vi "RSNRPZ Initialize Z5.vi"(8 "error in (no error)":errorcluster, 9 "Reset Device (T: Reset Device)":bool=TRUE, 10 "ID Query (T: Do Query)":bool=TRUE, 11 "Port (A)":i32(ring) items=["A", "B", "C", "D"]) -> (0 "error out":errorcluster, 2 "Function return value":i32, 3 "Instrument Handle":u32)   [LabVIEW 2010]
doc: "This VI performs the following initialization actions and assigned specified sesnor to channel 1:\n\n- Opens a session to the specified device using the interface and address specified in the Resource Name control.\n\n- Performs an identification query on the sensor.\n\n- Resets the instrument to a known state.\n\n- Sends initialization commands to the sensor\n\n- Returns an Instrument Handle which is used to differentiate between different sessions of this instrument driver."
uses:
  rsnrpz_32.dll
panel:
  # "Warning: The driver requires NRP Toolkit installed on your computer"
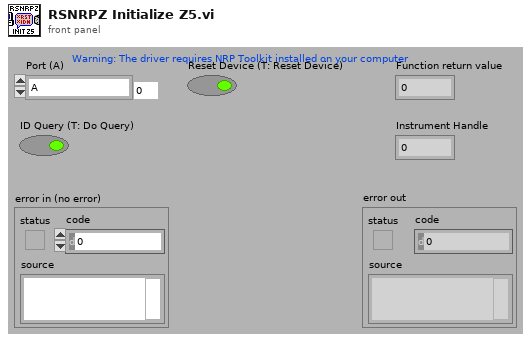
[diagram p1: front panel]
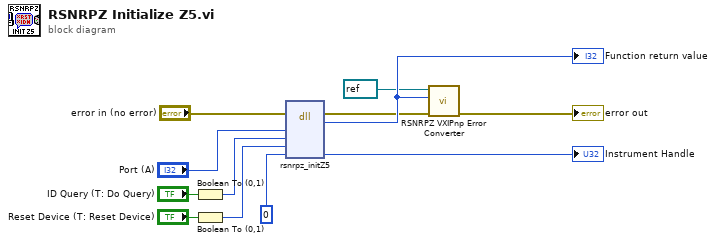
[diagram p0: block diagram]
diagram:
  n1 = Boolean To (0,1)(Boolean="ID Query (T: Do Query)") -> (0, 1=w8:i16)
  n2 = Boolean To (0,1)(Boolean="Reset Device (T: Reset Device)") -> (0, 1=w9:i16)
  n3 = dll-call lib="rsnrpz_32.dll" fn="rsnrpz_initZ5"(error in="error in (no error)", "Port"="Port (A)", "ID Query"=w8, "Reset Device"=w9, "Instrument Handle"=u32 0) -> (error out=w3:errorcluster, "return type"=w5:i32, "Instrument Handle"=→"Instrument Handle":u32)  [unwired: 5 in, 1 out]
  "Function return value" <- w5
  n4 = call <instrlib>:"RSNRPZ VXIPnp Error Converter.vi"("error in"=w3, "VXIPnp error code"=w5, "VISA session"=refnum<visa-resource-name> refnum) -> ("error out"=→"error out":errorcluster)  [unwired: 7 in, 1 out]
